vi "GenerateChangedFilesList.vi"(6 "GUI Mode? {F)":bool, 8 "error in (no error)":errorcluster) -> (0 "error out":errorcluster)   [LabVIEW 2023, in "CheckModifiedVIs.lvlib"]
uses:
  <vilib>/Hampel Software Engineering/Git API/Git API/GIT-api.lvclass/GIT-api.ctl
  <vilib>/Hampel Software Engineering/Git API/Git API/Accessors/GIT-Set Working Dir.vi
  CheckModifiedVIs.lvlib
  <vilib>/Hampel Software Engineering/Git API/Git API/GIT-api.lvclass
  <vilib>/Wiresmith Technology/G CLI/CLI Class/CLI.lvclass
  Reusables/Reusables.lvlib
panel:
  out "std out":string
  in  "Tab Control":T1(tab)
  in  "Output File Path":path=path "E:/sw-deps-monitor/changed-files.txt"
  in  "Branch 2":string="initial-ci-check-yml"
  in  "Branch 1":string="main"
  in  "Workspace Path":path=path "E:/sw-deps-monitor"
  out "Args":string[](array[string])=["E:\\sw-deps-monitor", "main", "initial-ci-check-yml", "E:\\sw-deps-monitor\\changed-files.txt"]
  # "When in GUI Mode, the controls will be used, \nin CLI Mode the Args will be used"
  # "Workspace Path"
  # "Branch 1"
  # "Branch 2"
  # "Output File Path"
  # "Command to run the VI from terminal\n\ng-cli -v --lv-ver 2023 --arch 32 \"E:\\sw-deps-monitor\\CICD\\Reusables\\GenerateChangedFilesList.vi\" \n-- \"E:\\sw-deps-monitor\" \"main\" \"initial-ci-check-yml\" \"E:\\sw-deps-monitor\\changed-files.txt\""
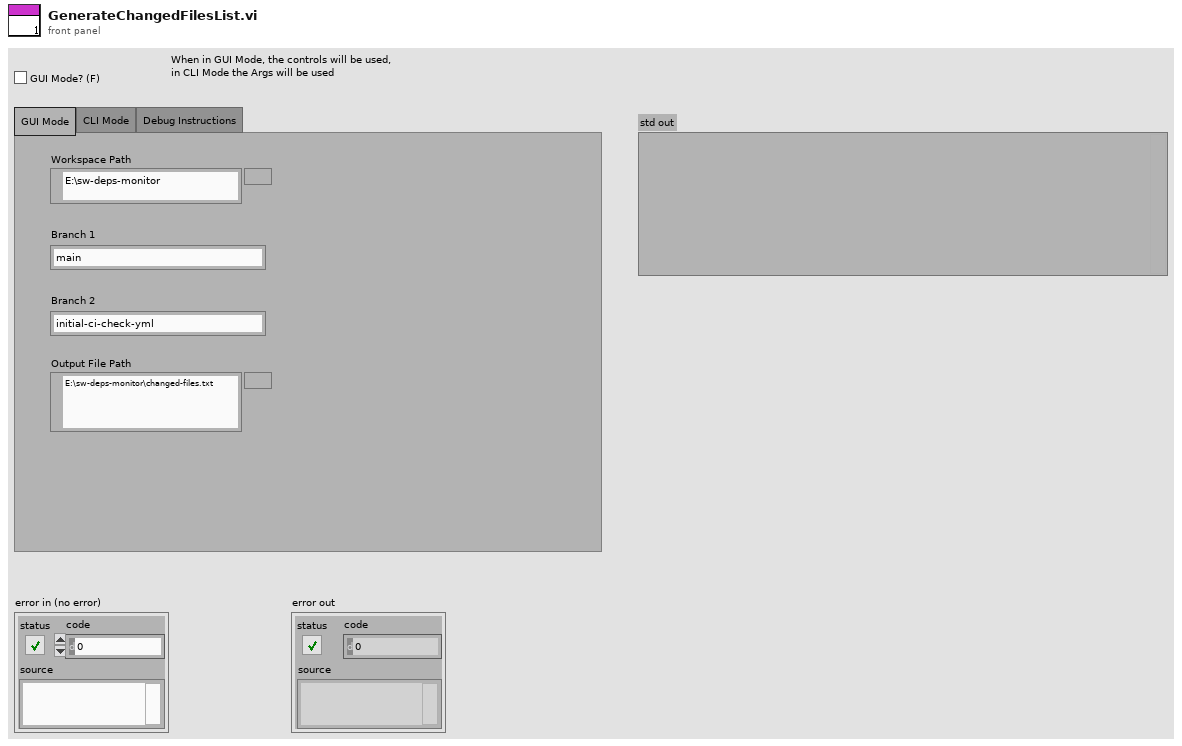
[diagram p1: front panel]
types:
  T1 = enum32{"GUI Mode", "CLI Mode", "Debug Instructions"}
  T2 = enum16{"open", "replace", "create", "open or create", "replace or create", "replace or create with confirmation"}
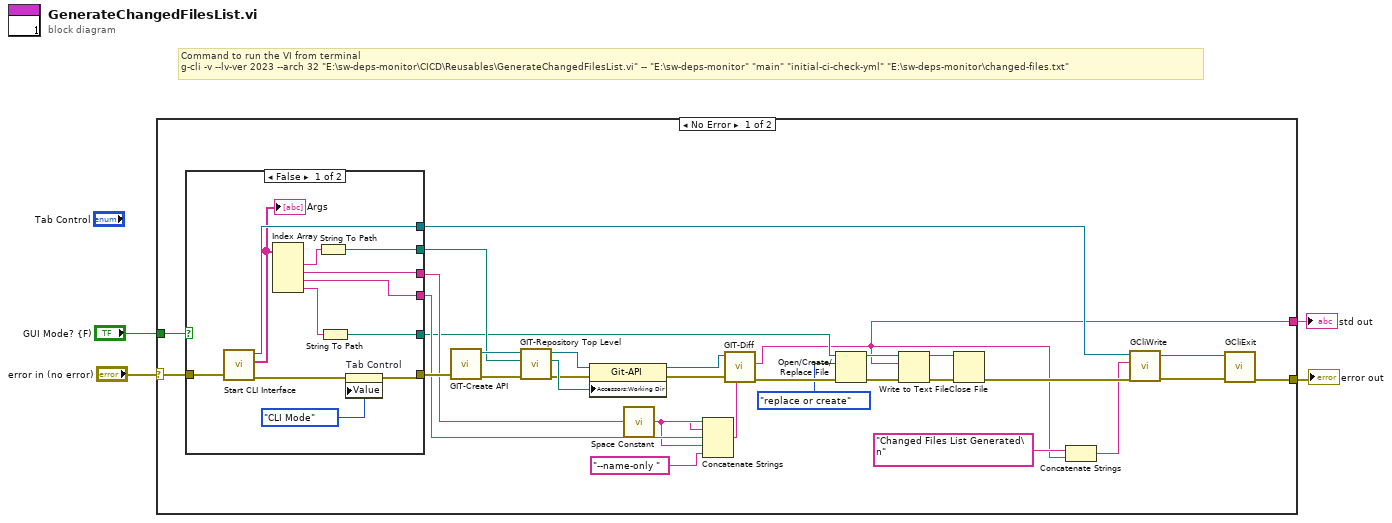
[diagram p0: block diagram]
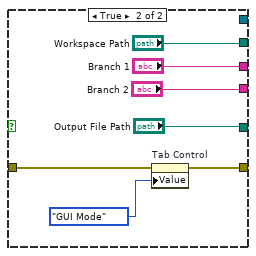
[diagram p2: hidden frame]
diagram:
  # "Command to run the VI from terminal\ng-cli -v --lv-ver 2023 --arch 32 \"E:\\sw-deps-monitor\\CICD\\Reusables\\GenerateChangedFilesList.vi\" -- \"E:\\sw-deps-monitor\" \"main\" \"initial-ci-check-yml\" \"E:\\sw-deps-monitor\\changed-files.txt\""
  n1 = case shown="No Error" "error in (no error)" {
    selector: "error in (no error)" -> [w25 w55]
    tunnel: "GUI Mode? {F)" -> [w26 _]
    tunnel: [w6 _] -> w2
    tunnel: [w9 w55] -> w1
    frame No Error {
      n2 = case shown="False" w26 {
        tunnel: [w46 "Branch 1"] -> w22
        tunnel: [w43 "Workspace Path"] -> w23
        tunnel: [w42 "Output File Path"] -> w18
        tunnel: [w45 "Branch 2"] -> w21
        tunnel: w25 -> [w41 w50]
        tunnel: [w38 w48] -> w24
        tunnel: [w40 _] -> w11
        frame False {
          n3 = call <vilib>:"Start CLI Interface.vi"("error in (no error)"=w41) -> ("error out"=w39:errorcluster, "Custom Parameters"=w36:string[], "CLI out"=w40:refnum<class "CLI.lvclass">)  [unwired: 7 in, 1 out]
          "Args" <- w36
          n4 = Index Array(array=w36) -> (element #1=w47:string, element #2=w46:string, element #3=w45:string, element #4=w44:string)  [unwired: 4 in]
          n5 = String To Path(string=w47) -> (path=w43:path)
          n6 = String To Path(string=w44) -> (path=w42:path)
          n7 = property on="Tab Control" class="TabCtl (strict)"(error in=w39, "Value"=enum32{"GUI Mode", "CLI Mode"}."CLI Mode" ("Tab Control")) -> (error out=w38:errorcluster)  [unwired: 1 in, 1 out]
        }
        frame True {
          n8 = property on="Tab Control" class="TabCtl (strict)"(error in=w50, "Value"=enum32{"GUI Mode", "CLI Mode"}."GUI Mode" ("Tab Control")) -> (error out=w48:errorcluster)  [unwired: 1 in, 1 out]
        }
      }
      n9 = call <vilib>:"GIT-Create API.vi"("error in"=w24) -> ("error out"=w31:errorcluster, "git-api out"=w34:refnum<class "GIT-api.lvclass">)  [unwired: 9 in]
      n10 = call <vilib>:"GIT-Repository Top Level.vi"("error in"=w31, "Current Path"=w23, "git-api in"=w34) -> ("error out"=w32:errorcluster, "Repo Top Level Path"=w33:path, "git-api out"=w35:refnum<class "GIT-api.lvclass">)  [unwired: 6 in]
      n11 = property class="Git-API"(reference=w35, error in=w32, "Accessors:Working Dir"=w33) -> (reference out=w29:refnum<class "GIT-api.lvclass">, error out=w30:errorcluster)
      n12 = call <vilib>:"Space Constant.vi"() -> ("String"=w20:string)
      n13 = Concatenate Strings(w22, w20, w21, w20, "--name-only " ("string")) -> (w28:string)
      n14 = call <vilib>:"GIT-Diff.vi"("param"=w28, "error in"=w30, "git-api in"=w29) -> ("error out"=w19:errorcluster, "std out"=w6:string)  [unwired: 6 in, 1 out]
      n15 = Open/Create/Replace File(file path (use dialog)=w18, error in=w19, operation (0:open)=T2."replace or create") -> (refnum out=w15:refnum<file>, error out=w16:errorcluster)  [unwired: 3 in, 1 out]
      n16 = Write to Text File(file (use dialog)=w15, text=w6, error in=w16) -> (refnum out=w13:refnum<file>, error out=w14:errorcluster)  [unwired: 1 in, 1 out]
      n17 = Close File(refnum=w13, error in=w14) -> (error out=w12:errorcluster)  [unwired: 1 out]
      n18 = Concatenate Strings("Changed Files List Generated\n" ("Text to Write"), w6) -> (w5:string)
      n19 = call "GCliWrite.vi"("error in (no error)"=w12, "Text to Write"=w5, "CLI in"=w11) -> ("error out"=w10:errorcluster, "CLI out"=w8:refnum<class "CLI.lvclass">)  [unwired: 7 in]
      n20 = call "GCliExit.vi"("error in (no error)"=w10, "CLI in"=w8) -> ("error out"=w9:errorcluster)  [unwired: 9 in]
    }
    frame Error {
    }
  }
  "error out" <- w1
  "std out" <- w2
